vi "RichToFlatgoogle_protobuf_Empty.vi"(5 "OutputClusterType":T1, 11 "InputCluster":T2) -> (3 "OutputCluster":T1)   [LabVIEW 2023, in "Generated_client.lvlib"]
uses:
  Generated_client.lvlib
  google_protobuf_Empty.ctl
  google_protobuf_Empty_Flat.ctl
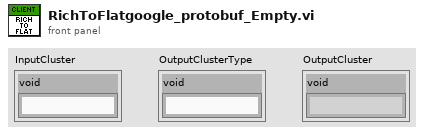
[diagram p1: front panel]
types:
  T1 = typedef "Generated_client.lvlib/google_protobuf_Empty_Flat.ctl" = cluster{"void":string}
  T2 = typedef "Generated_client.lvlib/google_protobuf_Empty.ctl" = cluster{"void":string}
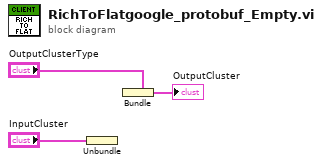
[diagram p0: block diagram]
diagram:
  n1 = Unbundle "Unbundle"("InputCluster") -> ()  [unwired: 1 out]
  n2 = Bundle "Bundle"(cluster="OutputClusterType") -> (→"OutputCluster":T1)  [unwired: 1 in]
